vi "Test Actor Methods.vi"() -> ()   [LabVIEW 2018, in "Acquisition.lvlib" / "Acquisition.lvclass"]
uses:
  Acquisition.lvclass
  Acquisition.lvclass/Acquisition.ctl
panel:
  out "error out":errorcluster
  out "Data":waveform(dbl)[](graph)
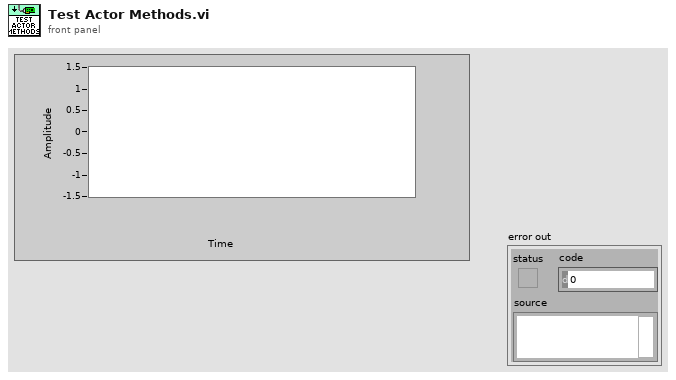
[diagram p1: front panel]
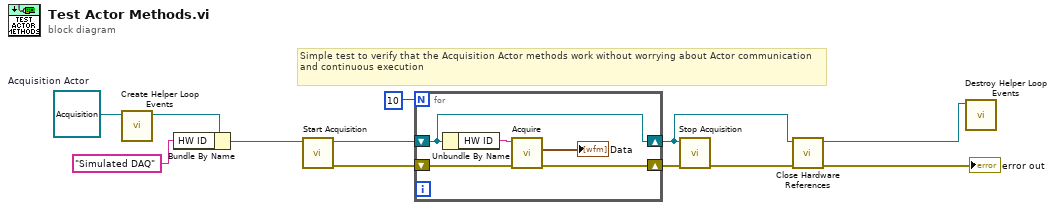
[diagram p0: block diagram]
diagram:
  w3 = refnum<class "Acquisition.lvclass"> refnum  # Acquisition Actor
  # "Simple test to verify that the Acquisition Actor methods work without worrying about Actor communication and continuous execution"
  n1 = call "Create Helper Loop Events.vi"("Acquisition in"=w3) -> ("Acquisition out"=w2:refnum<class "Acquisition.lvclass">)  [unwired: 10 in]
  n2 = Bundle By Name(cluster=w2, "HW ID"="Simulated DAQ") -> (w5:refnum<class "Acquisition.lvclass">)
  n3 = call-dynamic "Start Acquisition.vi"("Acquisition in"=w5) -> ("error out"=w10:errorcluster, "Acquisition out"=w11:refnum<class "Acquisition.lvclass">)  [unwired: 9 in]
  n4 = for {
    N: 10 -> [_]
    shift-right: [w15] -> w7
    shift-left: w11 -> [w15]
    shift-right: [w14] -> w9
    shift-left: w10 -> [w17]
    n5 = Unbundle By Name(w15) -> ("HW ID"=w16:string)
    n6 = call "Acquire.vi"("error in (no error)"=w17, "HW ID in"=w16) -> ("error out"=w14:errorcluster, "Graph Data"=→"Data":waveform(dbl)[])  [unwired: 7 in, 1 out]
  }
  n7 = call-dynamic "Stop Acquisition.vi"("error in (no error)"=w9, "Acquisition in"=w7) -> ("error out"=w8:errorcluster)  [unwired: 9 in]
  n8 = call-dynamic "Close Hardware References.vi"("error in (no error)"=w8, "Acquisition in"=w7) -> ("error out"=→"error out":errorcluster, "Acquisition out"=w1:refnum<class "Acquisition.lvclass">)  [unwired: 8 in]
  n9 = call "Destroy Helper Loop Events.vi"("Acquisition in"=w1) -> ()  [unwired: 11 in]
